vi "Add1 Value Change.vi"(11 "References":T1) -> (0 "error out":errorcluster)   [LabVIEW 2015, in "TDMS datalogger editor node.lvclass"]
uses:
  TDMS datalogger editor node.lvclass
  <vilib>/NI/DCAF/Tag Editor Core/Table API/Table Manager/object ref.ctl
  <vilib>/NI/DCAF/Tag Editor Core/Configuration Editor/Classes/Engine Parent/Engine Parent Editor Node.lvclass
  <vilib>/NI/DCAF/Tag Editor Core/Configuration Editor/Classes/Module editor node/module editor node.lvclass
  TDMS datalogger editor node.lvclass/TDMS datalogger editor node.ctl
  <vilib>/NI/DCAF/Tag Editor Core/Table API/Table Manager/Table Manager.lvclass
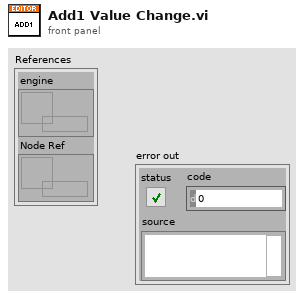
[diagram p1: front panel]
types:
  T1 = typedef "Table Manager.lvlib/Table Manager.lvclass/object ref.ctl" = cluster{"engine":refnum<data-value>, "Node Ref":refnum<data-value>}
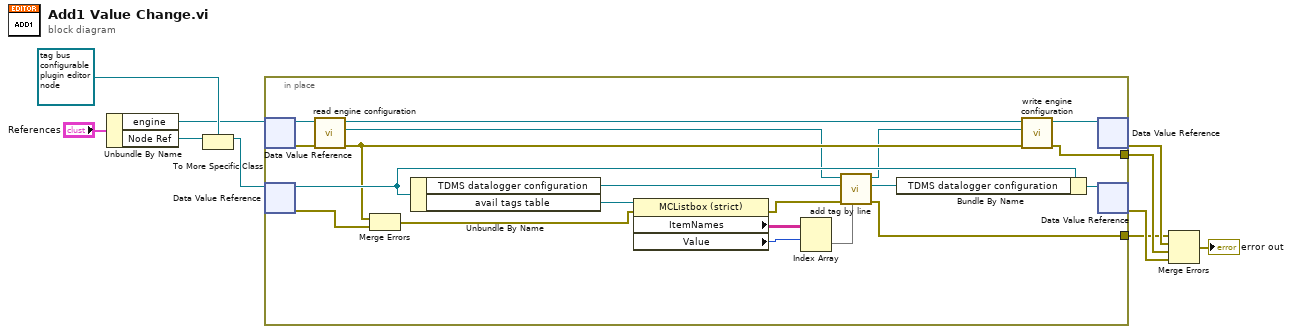
[diagram p0: block diagram]
diagram:
  n1 = Unbundle By Name("References") -> ("engine"=w3:refnum<data-value>, "Node Ref"=w5:refnum<data-value>)
  n2 = To More Specific Class(target class=refnum<data-value> refnum ("data value reference"), reference=w5) -> (specific class reference=w2:refnum<data-value>)  [unwired: 1 in, 1 out]
  n3 = in-place {
    in-place-border: [w16] -> w7
    in-place-border: [w24] -> w8
    n4 = in-place-dvr #1(w3) -> (w26:refnum<class "Engine Parent Editor Node.lvclass">, w27:errorcluster)
    n5 = in-place-dvr #2(w2) -> (w23:refnum<class "TDMS datalogger editor node.lvclass">, w29:errorcluster)
    n6 = call <vilib>:"read engine configuration.vi"("error in"=w27, "Engine Parent Editor Node in"=w26) -> ("error out"=w22:errorcluster, "engine configuration"=w14:refnum<class "engine configuration.lvclass">, "Engine Parent Editor Node out"=w25:refnum<class "Engine Parent Editor Node.lvclass">)  [unwired: 7 in]
    n7 = Merge Errors(w22, w29) -> (w13:errorcluster)
    n8 = Unbundle By Name(w23) -> ("TDMS datalogger configuration"=w18:refnum<class "TDMS datalogger configuration.lvclass">, "avail tags table"=w11:refnum<vi>)
    n9 = property on="Property Node" class="MCListbox (strict)"(reference=w11, error in=w13) -> (error out=w20:errorcluster, "ItemNames"=w19:string[][], "Value"=w12:i32)  [unwired: 1 out]
    n10 = Index Array(array=w19, index (row)=w12) -> (element=w21:string[])  [unwired: 1 in]
    n11 = call "add tag by line.vi"("ItemNames"=w21, "error in"=w20, "TDMS datalogger configuration in"=w18, "engine configuration in"=w14) -> ("error out"=w16:errorcluster, "TDMS datalogger configuration out"=w17:refnum<class "TDMS datalogger configuration.lvclass">, "engine configuration out"=w15:refnum<class "engine configuration.lvclass">)  [unwired: 5 in]
    n12 = Bundle By Name(cluster=w23, "TDMS datalogger configuration"=w17) -> (w30:refnum<class "TDMS datalogger editor node.lvclass">)
    n13 = call <vilib>:"write engine configuration.vi"("error in"=w22, "engine configuration"=w15, "Engine Parent Editor Node in"=w25) -> ("error out"=w24:errorcluster, "Engine Parent Editor Node out"=w28:refnum<class "Engine Parent Editor Node.lvclass">)  [unwired: 7 in]
    n14 = in-place-dvr #1(w28) -> (w9:errorcluster)  [unwired: 1 out]
    n15 = in-place-dvr #2(w30) -> (w10:errorcluster)  [unwired: 1 out]
  }
  n16 = Merge Errors(w7, w9, w8, w10) -> (→"error out":errorcluster)
